vi "solar_read ThisIni.vi"(8 "error in (no error)":errorcluster, 11 "solar in":refnum<class "solar.lvclass">) -> (0 "error out":errorcluster, 2 "Config Path":path, 3 "solar out":refnum<class "solar.lvclass">)   [LabVIEW 2018, in "solar.lvclass"]
doc: "This returns this target's configuration file path. The configuration directory is specified in the solar.ini file."
uses:
  solar.lvclass
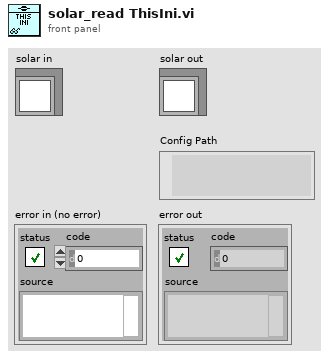
[diagram p1: front panel]
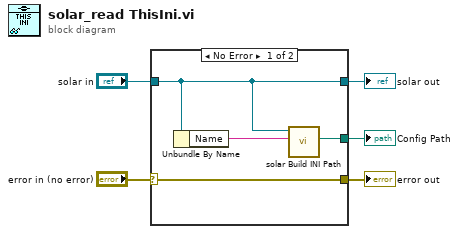
[diagram p0: block diagram]
diagram:
  n1 = case shown="No Error" "error in (no error)" {
    selector: "error in (no error)" -> [w9 w11]
    tunnel: "solar in" -> [w6 w10]
    tunnel: [w7 _] -> w4
    tunnel: [w9 w11] -> w3
    tunnel: [w6 w10] -> w1
    frame No Error {
      n2 = Unbundle By Name(w6) -> ("Name"=w8:string)
      n3 = call "solar Build INI Path.vi"("Name"=w8, "solar in"=w6) -> ("appended path"=w7:path)  [unwired: 8 in, 1 out]
    }
    frame Error {
    }
  }
  "error out" <- w3
  "solar out" <- w1
  "Config Path" <- w4
